vi "Swerve Go To.vi"(0 "Max Speed":dbl, 1 "Target X":dbl, 2 "Target Y":dbl, 3 "Target Angle":dbl) -> (6 "Done":bool)   [LabVIEW 2016]
uses:
  Robot Global Data.vi
  <vilib>/addons/control/pid/pid.llb/PID (DBL).vi
  <vilib>/addons/control/pid/NI_PID_pid.lvlib
  Apple Gyro/Apple Pi Gyro Library.lvlib
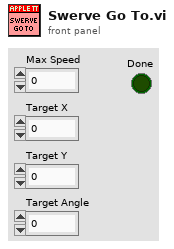
[diagram p1: front panel]
types:
  T1 = enum16{"Prepare to Rotate", "Rotate", "Prepare to Move", "Move"}
  T2 = cluster{"proportional gain (Kc)":dbl, "integral time (Ti, min)":dbl, "derivative time (Td, min)":dbl}
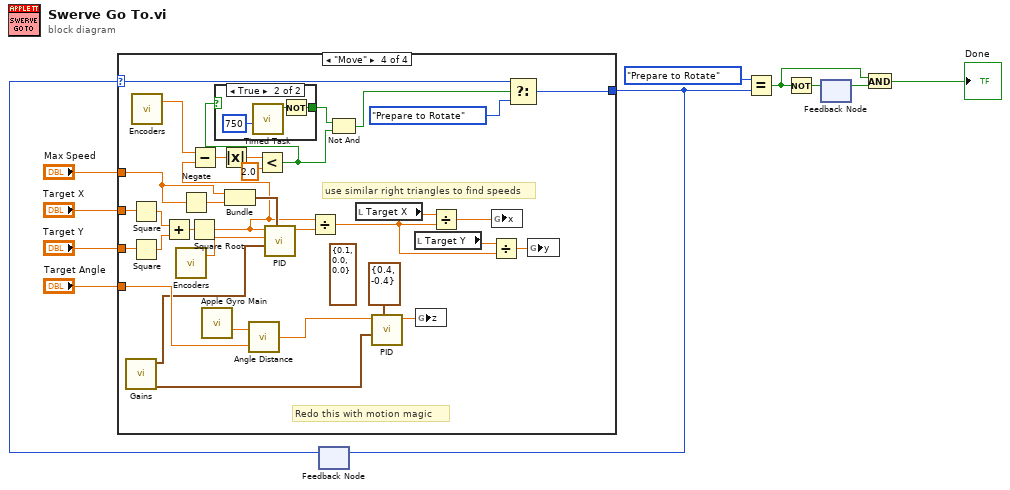
[diagram p0: block diagram]
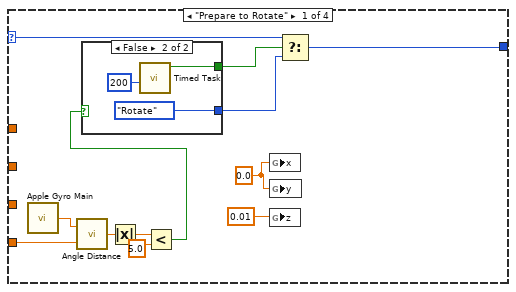
[diagram p2: hidden frame]
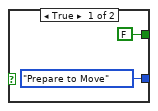
[diagram p3: hidden frame]
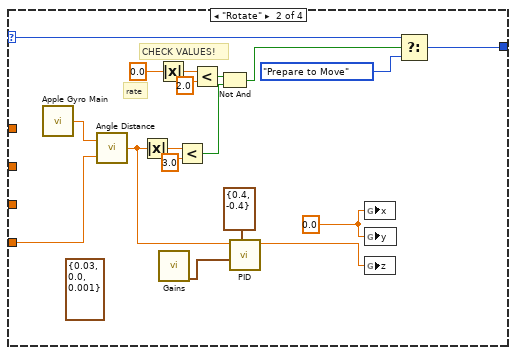
[diagram p4: hidden frame]
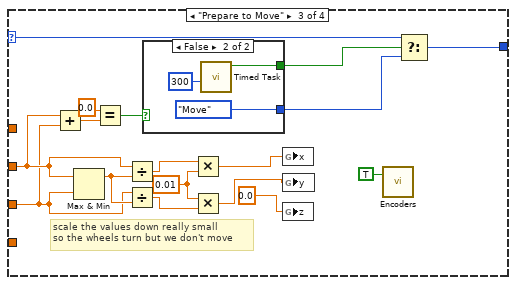
[diagram p5: hidden frame]
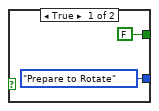
[diagram p6: hidden frame]
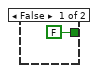
[diagram p7: hidden frame]
diagram:
  n1 = feedback #1() -> (w6:T1)  [unwired: 1 in]
  n2 = case shown="\"Move\"" w6 {
    selector: w6 -> [w22 w45 w62 w100]
    tunnel: [w23 w46 w63 w101] -> w1
    tunnel: "Target Angle" -> [w21 w35 _ w84]
    tunnel: "Target X" -> [_ _ w57 w98]
    tunnel: "Target Y" -> [_ _ w56 w97]
    tunnel: "Max Speed" -> [_ _ _ w91]
    frame "Prepare to Rotate" {
      w12 = 0.0
      n3 = call "Apple Gyro Main.vi"() -> ("Gyro Yaw Out"=w14:dbl)  [unwired: 4 in]
      n4 = call "Angle Distance.vi"("target angle"=w21, "current angle"=w14) -> ("distance"=w20:dbl)
      n5 = Absolute Value(x=w20) -> (abs(x)=w19:dbl)
      n6 = Less?(x=w19, y=5.0) -> (x < y?=w17:bool)
      n7 = case shown="False" w17 {
        tunnel: [FALSE w27] -> w15
        tunnel: [T1."Prepare to Move" T1."Rotate"] -> w16
        frame True {
        }
        frame False, Default {
          n8 = call "Timed Task.vi"("Time (ms)"=u32 200) -> ("Running"=w27:bool)  [unwired: 10 in]
        }
      }
      n9 = global write "Robot Global Data.vi" "x"(w12) -> ()
      n10 = global write "Robot Global Data.vi" "y"(w12) -> ()
      n11 = global write "Robot Global Data.vi" "z"(0.01) -> ()
      n12 = Select(t=w22, s=w15, f=w16) -> (s? t:f=w23:T1)
    }
    frame "Rotate" {
      (unwired) T2 {"proportional gain (Kc)"=0.03, "integral time (Ti, min)"=0.0, "derivative time (Td, min)"=0.001} ("PID gains")
      w29 = 0.0
      # "rate"
      # "CHECK VALUES!"
      n13 = call "Apple Gyro Main.vi"() -> ("Gyro Yaw Out"=w33:dbl)  [unwired: 4 in]
      n14 = call "Angle Distance.vi"("target angle"=w35, "current angle"=w33) -> ("distance"=w34:dbl)
      n15 = Absolute Value(x=w34) -> (abs(x)=w39:dbl)
      n16 = Absolute Value(x=0.0) -> (abs(x)=w42:dbl)
      n17 = call "Gains.vi"() -> ("Rot"=w31:T2)  [unwired: 10 in, 1 out]
      n18 = Less?(x=w39, y=3.0) -> (x < y?=w36:bool)
      n19 = Less?(x=w42, y=2.0) -> (x < y?=w38:bool)
      n20 = Not And(1:w36, 2:w38) -> (0:w37:bool)
      n21 = call-poly <vilib>:"PID.vi"("output range"=cluster{"output high":dbl, "output low":dbl} {"output high"=0.4, "output low"=-0.4}, "PID gains"=w31, "setpoint"=w34) -> ("output"=w30:dbl)  [unwired: 7 in, 1 out]
      n22 = global write "Robot Global Data.vi" "x"(w29) -> ()
      n23 = global write "Robot Global Data.vi" "y"(w29) -> ()
      n24 = global write "Robot Global Data.vi" "z"(w30) -> ()
      n25 = Select(t=w45, s=w37, f=T1."Prepare to Move") -> (s? t:f=w46:T1)
    }
    frame "Prepare to Move" {
      w60 = 0.01 ("y")
      # "scale the values down really small\nso the wheels turn but we don't move"
      n26 = Add(x=w57, y=w56) -> (x+y=w55:dbl)
      n27 = Max & Min(x=w57, y=w56) -> (max(x,y)=w61:dbl)  [unwired: 1 out]
      n28 = Equal?(x=0.0, y=w55) -> (x = y?=w53:bool)
      n29 = Divide(x=w57, y=w61) -> (x/y=w58:dbl)
      n30 = Divide(x=w56, y=w61) -> (x/y=w59:dbl)
      n31 = case shown="False" w53 {
        tunnel: [FALSE w67] -> w51
        tunnel: [T1."Prepare to Rotate" T1."Move"] -> w52
        frame True {
        }
        frame False, Default {
          n32 = call "Timed Task.vi"("Time (ms)"=u32 300) -> ("Running"=w67:bool)  [unwired: 10 in]
        }
      }
      n33 = Multiply(x=w58, y=w60) -> (x*y=w47:dbl)
      n34 = Multiply(x=w60, y=w59) -> (x*y=w48:dbl)
      n35 = global write "Robot Global Data.vi" "x"(w47) -> ()
      n36 = global write "Robot Global Data.vi" "y"(w48) -> ()
      n37 = global write "Robot Global Data.vi" "z"(0.0 ("Z")) -> ()
      n38 = call "Encoders.vi"("Reset All"=TRUE) -> ()  [unwired: 1 in, 2 out]
      n39 = Select(t=w62, s=w51, f=w52) -> (s? t:f=w63:T1)
    }
    frame "Move" {
      (unwired) T2 {"proportional gain (Kc)"=0.1, "integral time (Ti, min)"=0.0, "derivative time (Td, min)"=0.0} ("PID gains")
      # "Redo this with motion magic"
      # "use similar right triangles to find speeds"
      n40 = call "Gains.vi"() -> ("Rot"=w73:T2, "Drive"=w72:T2)  [unwired: 10 in]
      n41 = Square(x=w98) -> (x^2=w96:dbl)
      n42 = Square(x=w97) -> (x^2=w95:dbl)
      n43 = call "Encoders.vi"() -> ("Avg Absolute Distance"=w82:dbl)  [unwired: 2 in, 1 out]
      n44 = Add(x=w96, y=w95) -> (x+y=w94:dbl)
      n45 = call "Encoders.vi"() -> ("Avg Absolute Distance"=w85:dbl)  [unwired: 2 in, 1 out]
      n46 = Negate(x=w91) -> (-x=w92:dbl)
      n47 = Square Root(x=w94) -> (sqrt(x)=w79:dbl)
      n48 = Subtract(x=w82, y=w79) -> (x-y=w88:dbl)
      n49 = call "Apple Gyro Main.vi"() -> ("Gyro Yaw Out"=w81:dbl)  [unwired: 4 in]
      n50 = Absolute Value(x=w88) -> (abs(x)=w89:dbl)
      n51 = Bundle("Max Speed"=w91, w92) -> (w93:cluster{"Max Speed":dbl, dbl})  [unwired: 1 in]
      n52 = call "Angle Distance.vi"("target angle"=w84, "current angle"=w81) -> ("distance"=w83:dbl)
      n53 = Less?(x=w89, y=2.0) -> (x < y?=w74:bool)
      n54 = case shown="True" w74 {
        tunnel: [FALSE w104] -> w75
        frame False {
        }
        frame True {
          n55 = call "Timed Task.vi"("Time (ms)"=750) -> ("Running"=w105:bool)  [unwired: 10 in]
          n56 = Not(x=w105) -> (.not. x?=w104:bool)
        }
      }
      n57 = call-poly <vilib>:"PID.vi"("output range"=w93, "PID gains"=w72, "process variable"=w85, "setpoint"=w79) -> ("output"=w80:dbl)  [unwired: 6 in, 1 out]
      n58 = Divide(x=w79, y=w80) -> (x/y=w77:dbl)
      n59 = Not And(1:w74, 2:w75) -> (0:w87:bool)
      n60 = local read "Target X"() -> (w78:dbl)
      n61 = call-poly <vilib>:"PID.vi"("output range"=cluster{"output high":dbl, "output low":dbl} {"output high"=0.4, "output low"=-0.4}, "PID gains"=w73, "setpoint"=w83) -> ("output"=w71:dbl)  [unwired: 7 in, 1 out]
      n62 = local read "Target Y"() -> (w76:dbl)
      n63 = global write "Robot Global Data.vi" "z"(w71) -> ()
      n64 = Divide(x=w78, y=w77) -> (x/y=w69:dbl)
      n65 = Divide(x=w76, y=w77) -> (x/y=w70:dbl)
      n66 = global write "Robot Global Data.vi" "x"(w69) -> ()
      n67 = Select(t=w100, s=w87, f=T1."Prepare to Rotate") -> (s? t:f=w101:T1)
      n68 = global write "Robot Global Data.vi" "y"(w70) -> ()
    }
  }
  n69 = feedback-in #1(w1) -> ()
  n70 = Equal?(x=T1."Prepare to Rotate", y=w1) -> (x = y?=w2:bool)
  n71 = Not(x=w2) -> (.not. x?=w4:bool)
  n72 = feedback #2() -> (w3:bool)  [unwired: 1 in]
  n73 = feedback-in #2(w4) -> ()
  n74 = And(x=w2, y=w3) -> (x .and. y?=→"Done":bool)
